vi "Push Sample.vi"(8 "error in (no error)":errorcluster, 11 "cRIO-CO2 in":refnum<class "cRIO-CO2.lvclass">) -> (0 "error out":errorcluster, 3 "cRIO-CO2 out":refnum<class "cRIO-CO2.lvclass">)   [LabVIEW 2015, in "cRIO-Carbondioxide.lvlib" / "cRIO-CO2.lvlib" / "cRIO-CO2.lvclass"]
uses:
  cRIO-CO2.lvclass
  cRIO-CO2.lvclass/cRIO-CO2.ctl
  Controls/Sample Push State Enumerator.ctl
  cRIO-CO2 Messages/Sample Push Reset to Idle Msg/Sample Push Reset to Idle Msg.lvclass/Sample Push Reset to Idle Msg.ctl
  <vilib>/ActorFramework/Message Enqueuer/Message Enqueuer.lvclass/Message Enqueuer.ctl
  Controls/Sample Transfer Container Enumerator.ctl
  Blowers Heaters Enumerator.ctl
  Controls/Sample Transfer State Enumerator.ctl
  <vilib>/ActorFramework/Time-Delayed Send Message/Time-Delay Override Options.ctl
  <vilib>/ActorFramework/Message Enqueuer/Enqueue.vi
  State Elapsed Time.vi
  <vilib>/ActorFramework/Message Priority Queue/Priority Enqueue.vi
  cRIO-CO2 Messages/Sample Push Reset to Idle Msg/Sample Push Reset to Idle Msg.lvclass
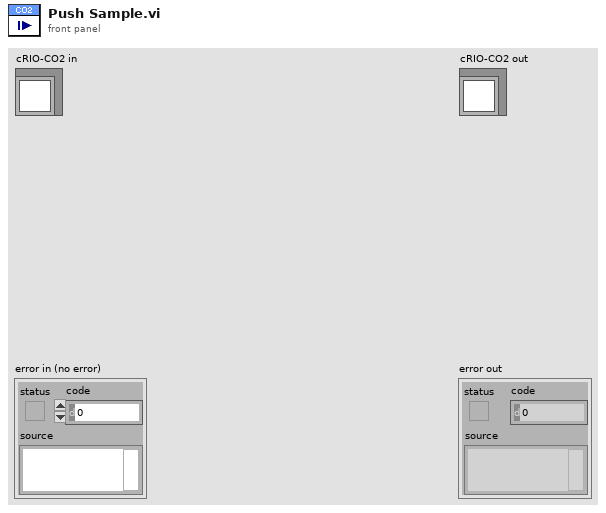
[diagram p1: front panel]
types:
  T1 = typedef "Sample Push State Enumerator.ctl" = enum16{"Undefined", "Initialize", "Dilute", "Close Transfer Line", "Start Heaters", "Warm Up Syringe", "Ready to Push", "Push", "Initiate Stash", "Stash", "Complete", "Abort", "Idle", "Error"}
  T2 = typedef "Sample Transfer Container Enumerator.ctl" = enum16{"None", "Sample 1", "Sample 2", "Sample 3", "Sample 4", "Sample 5", "Storage 01", "Storage 02", "Storage 03", "Storage 04", "Storage 05", "Storage 06", "Storage 07", "Storage 08", "Storage 09", "Storage 10", "Storage 11", "Storage 12", "Syringe", "Undefined"}
  T3 = typedef "cRIO-Carbondioxide.lvlib/cRIO-CO2.lvlib/cRIO-CO2.lvclass/Blowers Heaters Enumerator.ctl" = enum16{"Tank Blower 1", "Tank Blower 2", "Tank Blower 3", "Tank Blower 4", "Syringe Blower", "Syringe Heater", "Piston Heater", "Undefined"}
  T4 = typedef "Sample Transfer State Enumerator.ctl" = enum16{"Idle", "Initialize", "Check Containers", "Check Temperatures", "Start Turbo", "Warm Up Containers", "Prepare for purging", "Purge Capillary", "Purge", "Open Containers", "Introduce Sample", "Measure Base Pressure", "Home Syringe", "Start Freezer", "Freeze Target", "Crystalize", "Initiate Stash", "Stash", "Polish", "Stop Freezers", "Push Sample", "Complete", "Abort", "Error", "Undefined"}
  T5 = typedef "Time-Delay Override Options.ctl" = enum16{"Send next copy now", "Skip next scheduled copy", "Send next copy now and stop all further copies", "Stop all further copies"}
  T6 = typedef "Vacuum State Enumerator.ctl" = enum16{"Pressure Rising", "Plateau", "Pressure Dropping", "Valley", "Low Valley", "Leak", "Unknown"}
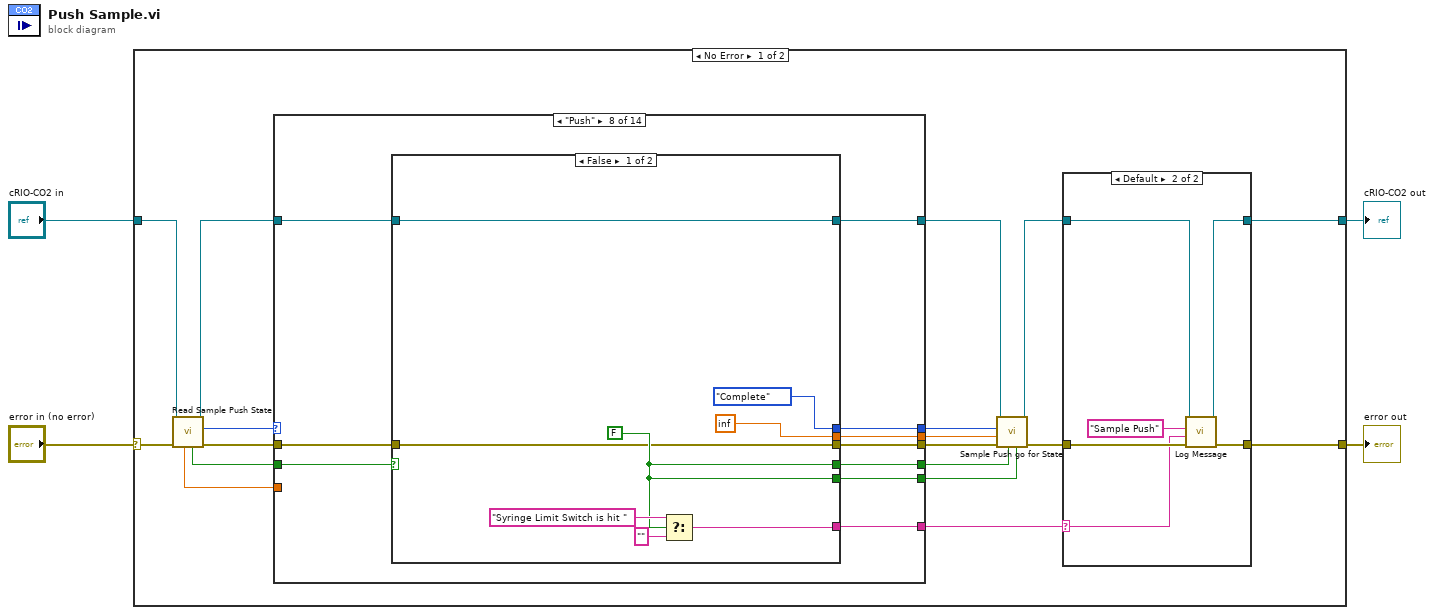
[diagram p0: block diagram]
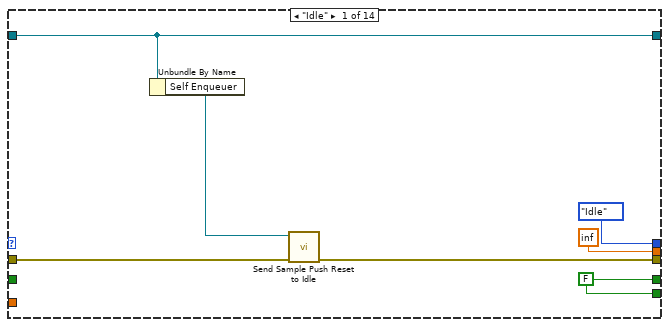
[diagram p3: hidden frame]
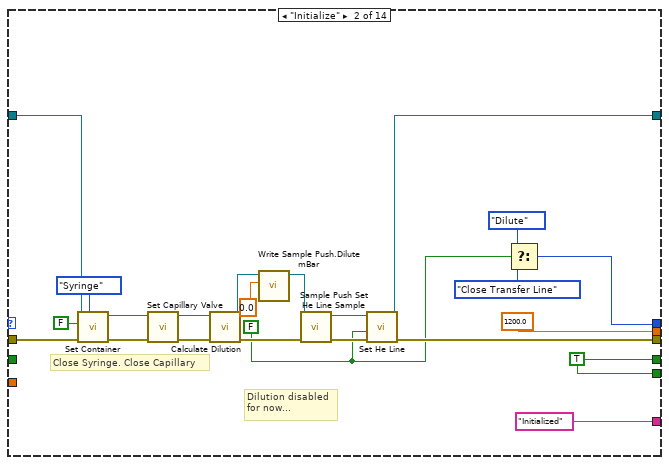
[diagram p4: hidden frame]
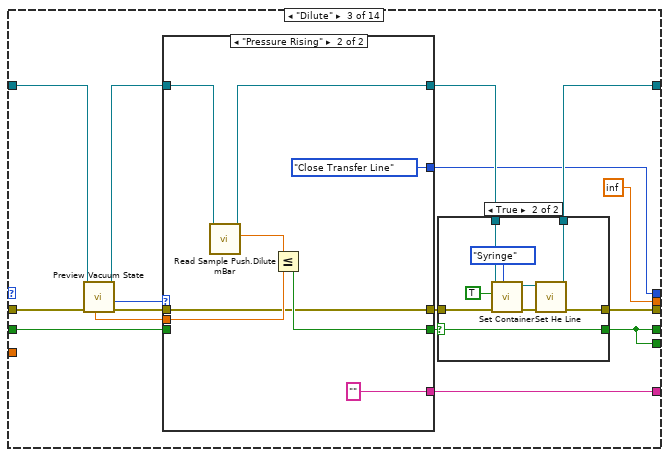
[diagram p5: hidden frame]
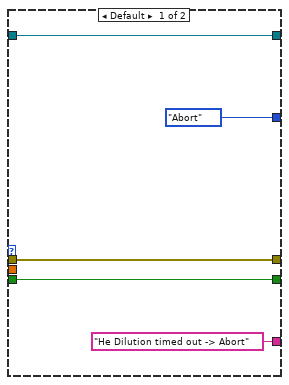
[diagram p7: hidden frame]
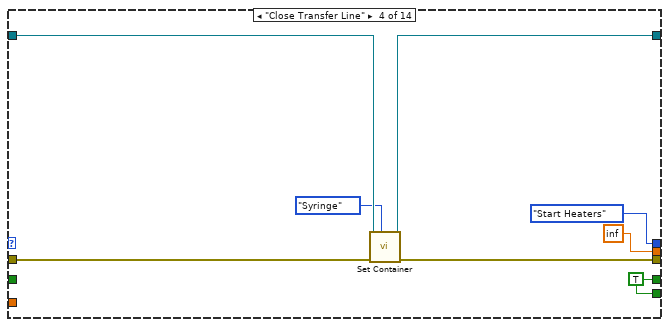
[diagram p8: hidden frame]
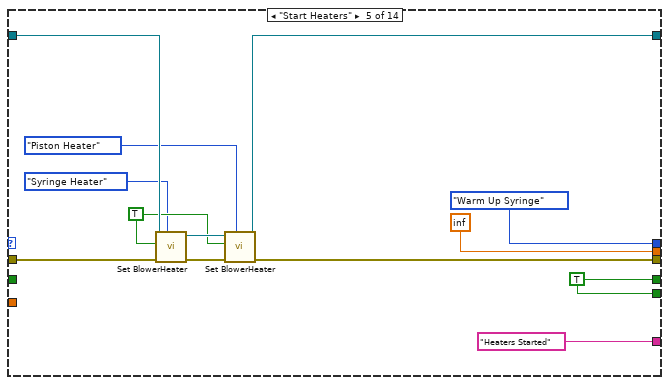
[diagram p9: hidden frame]
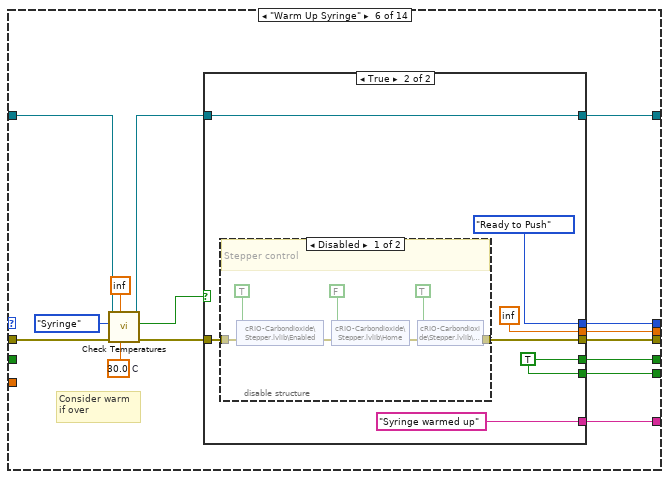
[diagram p10: hidden frame]
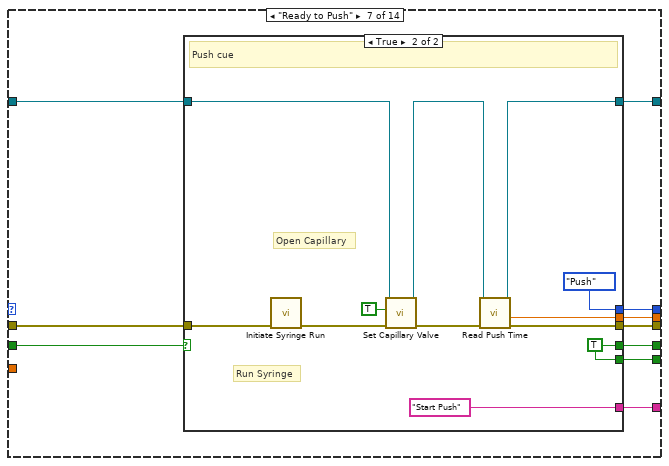
[diagram p13: hidden frame]
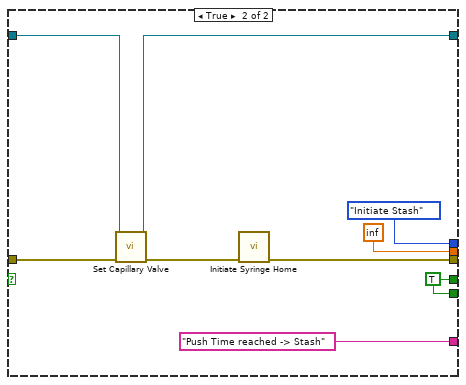
[diagram p15: hidden frame]
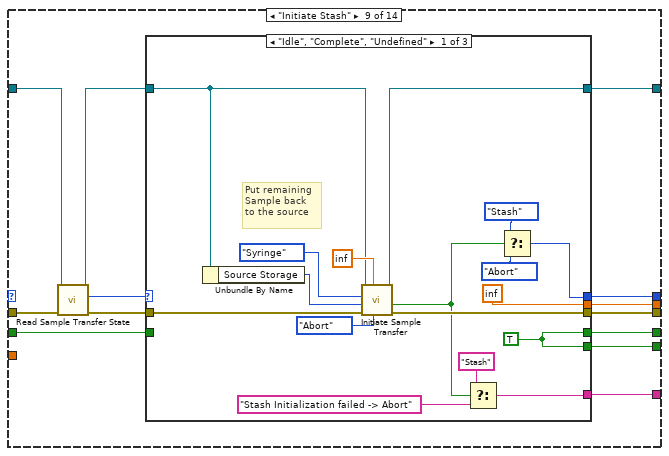
[diagram p16: hidden frame]
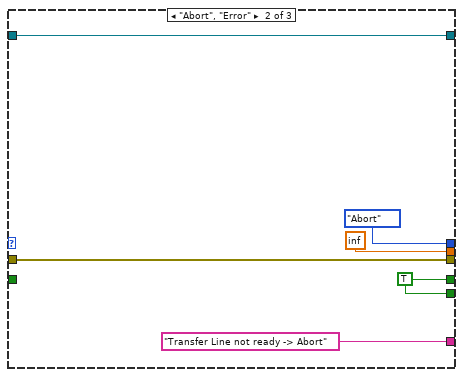
[diagram p17: hidden frame]
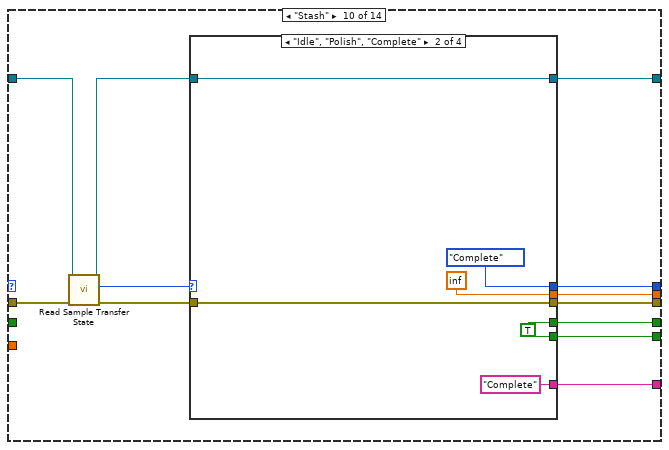
[diagram p19: hidden frame]
diagram:
  n1 = case shown="No Error" "error in (no error)" {
    selector: "error in (no error)" -> [w22 w326]
    tunnel: [w17 w326] -> w3
    tunnel: [w16 w325] -> w1
    tunnel: "cRIO-CO2 in" -> [w21 w325]
    frame No Error {
      n2 = call "Read Sample Push State.vi"("error in (no error)"=w22, "cRIO-CO2 in"=w21) -> ("error out"=w20:errorcluster, "Sample Push State"=w18:T1, "cRIO-CO2 out"=w19:refnum<class "cRIO-CO2.lvclass">, "Timeout?"=w14:bool, "Elapsed Time (s)"=w6:dbl)  [unwired: 3 in, 2 out]
      n3 = case shown="\"Push\"" w18 {
        tunnel: w20 -> [w34 w59 w75 w106 w122 w130 w155 w179 w218 w255 w287 w297 w308 w323]
        tunnel: [w31 w50 w67 w105 w112 w136 w162 w186 w213 w249 w277 w299 w314 w323] -> w13
        tunnel: w19 -> [w32 w57 w74 w104 w121 w126 w164 w188 w217 w254 w286 w296 w306 w324]
        tunnel: [_ "Initialized" ("String") w62 _ "Heaters Started" ("String") w135 w161 w185 w207 w244 "Complete" ("String") "Aborted" ("String") "Error" ("String") _] -> w15
        tunnel: w14 -> [_ _ w69 _ _ _ w156 w184 w206 _ _ _ _ _]
        tunnel: [w37 w54 w63 w107 w111 w132 w160 w183 w210 w246 w283 FALSE ("Publish? (T)") FALSE ("Publish? (T)") w321] -> w10
        tunnel: [w37 w54 w63 w107 w111 w131 w157 w180 w209 w245 w282 FALSE ("Publish? (T)") FALSE ("Publish? (T)") w321] -> w9
        tunnel: [Sample_Push_State_Enumerator."Idle" ("Sample Push State") w41 w61 Sample_Push_State_Enumerator."Start Heaters" ("Sample Push State") Sample_Push_State_Enumerator."Warm Up Syringe" ("Sample Push State") w133 w159 w182 w212 w248 Sample_Push_State_Enumerator."Idle" ("Sample Push State") Sample_Push_State_Enumerator."Idle" ("Sample Push State") Sample_Push_State_Enumerator."Idle" ("Sample Push State") Sample_Push_State_Enumerator."Idle" ("Sample Push State")] -> w8
        tunnel: [inf ("State Timeout (Inf=no timeout )") 1200.0 ("State Timeout (Inf=no timeout )") inf ("State Timeout (Inf=no timeout )") inf ("State Timeout (Inf=no timeout )") inf ("State Timeout (Inf=no timeout )") w134 w158 w181 w211 w247 inf ("State Timeout (Inf=no timeout )") inf ("State Timeout (Inf=no timeout )") inf ("State Timeout (Inf=no timeout )") inf ("State Timeout (Inf=no timeout )")] -> w7
        tunnel: w6 -> [_ _ _ _ _ _ _ _ _ _ _ _ _ _]
        tunnel: [w32 w49 w65 w103 w113 w137 w163 w187 w215 w252 w278 w298 w313 w324] -> w5
        frame "Idle" {
          w37 = FALSE ("Publish? (T)")
          n4 = Unbundle By Name(w32) -> ("Self Enqueuer"=w33:refnum<class "Message Enqueuer.lvclass">)
          n5 = call "Send Sample Push Reset to Idle.vi"("error in (no error)"=w34, "Message Enqueuer"=w33) -> ("error out"=w31:errorcluster)  [unwired: 8 in, 1 out]
        }
        frame "Initialize" {
          w39 = FALSE ("Open/Close (Close)")
          w54 = TRUE ("Publish? (T)")
          # "Dilution disabled\nfor now..."
          # "Close Syringe. Close Capillary"
          n6 = call "Set Container.vi"("Container"=Sample_Transfer_Container_Enumerator."Syringe", "error in (no error)"=w59, "Open/Close (Close)"=FALSE, "cRIO-CO2 in"=w57) -> ("error out"=w56:errorcluster, "cRIO-CO2 out"=w55:refnum<class "cRIO-CO2.lvclass">)  [unwired: 6 in]
          n7 = call "Set Capillary Valve.vi"("error in (no error)"=w56, "cRIO-CO2 in"=w55) -> ("error out"=w52:errorcluster, "cRIO-CO2 out"=w51:refnum<class "cRIO-CO2.lvclass">)  [unwired: 8 in]
          n8 = call "Calculate Dilution.vi"("error in (no error)"=w52, "cRIO-CO2 in"=w51) -> ("error out"=w47:errorcluster, "cRIO-CO2 out"=w48:refnum<class "cRIO-CO2.lvclass">)  [unwired: 6 in, 2 out]
          n9 = call "Write Sample Push.Dilute mBar.vi"("Dilute mBar"=0.0, "cRIO-CO2 in"=w48) -> ("cRIO-CO2 out"=w45:refnum<class "cRIO-CO2.lvclass">)  [unwired: 9 in]
          n10 = call "Sample Push Set He Line Sample.vi"("error in (no error)"=w47, "cRIO-CO2 in"=w45) -> ("error out"=w46:errorcluster, "cRIO-CO2 out"=w44:refnum<class "cRIO-CO2.lvclass">)  [unwired: 8 in]
          n11 = call "Set He Line.vi"("error in (no error)"=w46, "Open/Close (Close)"=w39, "cRIO-CO2 in"=w44) -> ("error out"=w50:errorcluster, "cRIO-CO2 out"=w49:refnum<class "cRIO-CO2.lvclass">)  [unwired: 7 in]
          n12 = Select(t=Sample_Push_State_Enumerator."Dilute" ("Sample Push State"), s=w39, f=Sample_Push_State_Enumerator."Close Transfer Line" ("Sample Push State")) -> (s? t:f=w41:T1)
        }
        frame "Dilute" {
          n13 = call "Preview Vacuum State.vi"("error in (no error)"=w75, "cRIO-CO2 in"=w74) -> ("error out"=w71:errorcluster, "State"=w73:T6, "cRIO-CO2 out"=w72:refnum<class "cRIO-CO2.lvclass">, "Raw Pressure"=w70:dbl)  [unwired: 3 in, 3 out]
          n14 = case shown="\"Pressure Rising\"" w73 {
            tunnel: w72 -> [w92 w99]
            tunnel: w71 -> [w93 w97]
            tunnel: w70 -> [_ w100]
            tunnel: w69 -> [w91 _]
            tunnel: [w93 w97] -> w68
            tunnel: [w91 w98] -> w64
            tunnel: [w92 w96] -> w66
            tunnel: ["He Dilution timed out -> Abort" ("String") "" ("String")] -> w62
            tunnel: [Sample_Push_State_Enumerator."Abort" ("Sample Push State") Sample_Push_State_Enumerator."Close Transfer Line" ("Sample Push State")] -> w61
            frame Default {
            }
            frame "Pressure Rising" {
              n15 = call "Read Sample Push.Dilute mBar.vi"("cRIO-CO2 in"=w99) -> ("Dilute mBar"=w101:dbl, "cRIO-CO2 out"=w96:refnum<class "cRIO-CO2.lvclass">)  [unwired: 9 in]
              n16 = Less Or Equal?(x=w101, y=w100) -> (x <= y?=w98:bool)
            }
          }
          n17 = case shown="True" w64 {
            selector: w64 -> [w78 w86]
            tunnel: w68 -> [w79 w85]
            tunnel: [w79 w88] -> w67
            tunnel: w66 -> [w77 w82]
            tunnel: [w77 w87] -> w65
            tunnel: [w78 w86] -> w63
            frame False {
            }
            frame True {
              n18 = call "Set Container.vi"("Container"=Sample_Transfer_Container_Enumerator."Syringe", "error in (no error)"=w85, "Open/Close (Close)"=TRUE, "cRIO-CO2 in"=w82) -> ("error out"=w84:errorcluster, "cRIO-CO2 out"=w83:refnum<class "cRIO-CO2.lvclass">)  [unwired: 6 in]
              n19 = call "Set He Line.vi"("error in (no error)"=w84, "cRIO-CO2 in"=w83) -> ("error out"=w88:errorcluster, "cRIO-CO2 out"=w87:refnum<class "cRIO-CO2.lvclass">)  [unwired: 8 in]
            }
          }
        }
        frame "Close Transfer Line" {
          w107 = TRUE ("Publish? (T)")
          n20 = call "Set Container.vi"("Container"=Sample_Transfer_Container_Enumerator."Syringe", "error in (no error)"=w106, "cRIO-CO2 in"=w104) -> ("error out"=w105:errorcluster, "cRIO-CO2 out"=w103:refnum<class "cRIO-CO2.lvclass">)  [unwired: 7 in]
        }
        frame "Start Heaters" {
          w111 = TRUE ("Publish? (T)")
          w118 = TRUE ("ON/OFF (OFF)")
          n21 = call "Set BlowerHeater.vi"("Blower/Heater"=Blowers_Heaters_Enumerator."Syringe Heater", "error in (no error)"=w122, "ON/OFF (OFF)"=w118, "cRIO-CO2 in"=w121) -> ("error out"=w120:errorcluster, "cRIO-CO2 out"=w119:refnum<class "cRIO-CO2.lvclass">)  [unwired: 6 in]
          n22 = call "Set BlowerHeater.vi"("Blower/Heater"=Blowers_Heaters_Enumerator."Piston Heater", "error in (no error)"=w120, "ON/OFF (OFF)"=w118, "cRIO-CO2 in"=w119) -> ("error out"=w112:errorcluster, "cRIO-CO2 out"=w113:refnum<class "cRIO-CO2.lvclass">)  [unwired: 6 in]
        }
        frame "Warm Up Syringe" {
          w128 = 30.0  # C
          # "Consider warm\nif over"
          n23 = call "Check Temperatures.vi"("lower limit (10C)"=w128, "upper limit (100C)"=inf, "error in (no error)"=w130, "Container"=Sample_Transfer_Container_Enumerator."Syringe", "cRIO-CO2 in"=w126) -> ("error out"=w129:errorcluster, "In Range?"=w124:bool, "cRIO-CO2 out"=w125:refnum<class "cRIO-CO2.lvclass">)  [unwired: 4 in]
          n24 = case shown="True" w124 {
            tunnel: w125 -> [w139 w143]
            tunnel: [w139 w143] -> w137
            tunnel: w129 -> [w138 w145]
            tunnel: [w138 w144] -> w136
            tunnel: [_ "Syringe warmed up"] -> w135
            tunnel: [_ inf ("State Timeout (Inf=no timeout )")] -> w134
            tunnel: [_ Sample_Push_State_Enumerator."Ready to Push" ("Sample Push State")] -> w133
            tunnel: [_ w141] -> w132
            tunnel: [_ w141] -> w131
            frame False {
            }
            frame True {
              w141 = TRUE
              n25 = disable-structure shown="Disabled" {
                disable-tunnel: w145 -> [w153 w154]
                disable-tunnel: [w151 w154] -> w144
                frame Disabled {
                  # "Stepper control"
                  n26 = shared-variable "cRIO-Carbondioxide\\Stepper.lvlib\\Enabled"(TRUE ("Enabled"), error in=w153) -> (error out=w150:errorcluster)
                  n27 = shared-variable "cRIO-Carbondioxide\\Stepper.lvlib\\Home"(FALSE ("Home"), error in=w150) -> (error out=w149:errorcluster)
                  n28 = shared-variable "cRIO-Carbondioxide\\Stepper.lvlib\\Run"(TRUE ("Run"), error in=w149) -> (error out=w151:errorcluster)
                }
                frame Enabled {
                }
              }
            }
          }
        }
        frame "Ready to Push" {
          n29 = case shown="True" w156 {
            tunnel: w164 -> [w166 w175]
            tunnel: [w166 w167] -> w163
            tunnel: [w165 w170] -> w162
            tunnel: [_ "Start Push"] -> w161
            tunnel: w155 -> [w165 w173]
            tunnel: [_ w176] -> w160
            tunnel: [_ Sample_Push_State_Enumerator."Push" ("Sample Push State")] -> w159
            tunnel: [_ w169] -> w158
            tunnel: [_ w176] -> w157
            frame False {
              # "Waiting for the Push Cue (Timeout cleared)"
            }
            frame True {
              w176 = TRUE ("Timeout?")
              # "Run Syringe"
              # "Open Capillary"
              # "Push cue"
              n30 = call "Initiate Syringe Run.vi"("error in (no error)"=w173) -> ("error out"=w172:errorcluster)  [unwired: 10 in]
              n31 = call "Set Capillary Valve.vi"("error in (no error)"=w172, "ON/OFF(OFF)"=TRUE, "cRIO-CO2 in"=w175) -> ("error out"=w171:errorcluster, "cRIO-CO2 out"=w168:refnum<class "cRIO-CO2.lvclass">)  [unwired: 7 in]
              n32 = call "Read Push Time.vi"("error in (no error)"=w171, "cRIO-CO2 in"=w168) -> ("error out"=w170:errorcluster, "Push Time (sec)"=w169:dbl, "cRIO-CO2 out"=w167:refnum<class "cRIO-CO2.lvclass">)  [unwired: 7 in]
            }
          }
        }
        frame "Push" {
          n33 = case shown="False" w184 {
            tunnel: w188 -> [w196 w200]
            tunnel: [w196 w199] -> w187
            tunnel: [w189 w197] -> w186
            tunnel: [w193 "Push Time reached -> Stash"] -> w185
            tunnel: w179 -> [w189 w201]
            tunnel: [w190 w204] -> w183
            tunnel: [Sample_Push_State_Enumerator."Complete" ("Sample Push State") Sample_Push_State_Enumerator."Initiate Stash" ("Sample Push State")] -> w182
            tunnel: [inf inf] -> w181
            tunnel: [w190 w204] -> w180
            frame False {
              w190 = FALSE
              n34 = Select(t="Syringe Limit Switch is hit ", s=w190, f="") -> (s? t:f=w193:string)
            }
            frame True {
              w204 = TRUE ("Timeout?")
              n35 = call "Set Capillary Valve.vi"("error in (no error)"=w201, "cRIO-CO2 in"=w200) -> ("error out"=w198:errorcluster, "cRIO-CO2 out"=w199:refnum<class "cRIO-CO2.lvclass">)  [unwired: 8 in]
              n36 = call "Initiate Syringe Home.vi"("error in (no error)"=w198) -> ("error out"=w197:errorcluster)  [unwired: 10 in]
            }
          }
        }
        frame "Initiate Stash" {
          n37 = call "Read Sample Transfer State.vi"("error in (no error)"=w218, "cRIO-CO2 in"=w217) -> ("error out"=w214:errorcluster, "Sample Transfer State"=w208:T4, "cRIO-CO2 out"=w216:refnum<class "cRIO-CO2.lvclass">)  [unwired: 4 in, 3 out]
          n38 = case shown="\"Idle\", \"Complete\", \"Undefined\"" w208 {
            tunnel: w216 -> [w231 w241 w243]
            tunnel: [w233 w241 w243] -> w215
            tunnel: w214 -> [w234 w240 w242]
            tunnel: [w228 w240 w242] -> w213
            tunnel: [w223 Sample_Push_State_Enumerator."Abort" ("Sample Push State") _] -> w212
            tunnel: [inf ("State Timeout (Inf=no timeout )") inf ("State Timeout (Inf=no timeout )") _] -> w211
            tunnel: [w227 w237 _] -> w210
            tunnel: [w227 w237 _] -> w209
            tunnel: [w222 "Transfer Line not ready -> Abort" _] -> w207
            tunnel: w206 -> [_ _ _]
            frame "Idle", "Complete", "Undefined" {
              w227 = TRUE
              # "Put remaining\nSample back\nto the source"
              n39 = Unbundle By Name(w231) -> ("Source Storage"=w229:T2)
              n40 = call "Initiate Sample Transfer.vi"("Fail State (Idle)"=Sample_Transfer_State_Enumerator."Abort", "Transfer mBar"=inf, "error in (no error)"=w234, "Target Container"=w229, "Source Container"=Sample_Transfer_Container_Enumerator."Syringe", "cRIO-CO2 in"=w231) -> ("error out"=w228:errorcluster, "Success?"=w220:bool, "cRIO-CO2 out"=w233:refnum<class "cRIO-CO2.lvclass">)  [unwired: 3 in]
              n41 = Select(t="Stash", s=w220, f="Stash Initialization failed -> Abort" ("t")) -> (s? t:f=w222:string)
              n42 = Select(t=Sample_Push_State_Enumerator."Stash", s=w220, f=Sample_Push_State_Enumerator."Abort" ("Sample Push State")) -> (s? t:f=w223:T1)
            }
            frame "Abort", "Error" {
              w237 = TRUE
            }
            frame Default {
            }
          }
        }
        frame "Stash" {
          n43 = call "Read Sample Transfer State.vi"("error in (no error)"=w255, "cRIO-CO2 in"=w254) -> ("error out"=w250:errorcluster, "Sample Transfer State"=w253:T4, "cRIO-CO2 out"=w251:refnum<class "cRIO-CO2.lvclass">)  [unwired: 4 in, 3 out]
          n44 = case shown="\"Idle\", \"Polish\", \"Complete\"" w253 {
            tunnel: [w257 w263 w269 w275] -> w252
            tunnel: w251 -> [w257 w263 w269 w275]
            tunnel: w250 -> [w256 w258 w268 w274]
            tunnel: [w256 w258 w268 w274] -> w249
            tunnel: [_ Sample_Push_State_Enumerator."Complete" ("Sample Push State") Sample_Push_State_Enumerator."Abort" ("Sample Push State") Sample_Push_State_Enumerator."Abort" ("Sample Push State")] -> w248
            tunnel: [_ inf inf inf] -> w247
            tunnel: [_ w260 w265 w271] -> w246
            tunnel: [_ w260 w265 w271] -> w245
            tunnel: [_ "Complete" "Transfer Error -> Abort" "Transfer Aborted -> Abort"] -> w244
            frame Default {
            }
            frame "Idle", "Polish", "Complete" {
              w260 = TRUE
            }
            frame "Error" {
              w265 = TRUE
            }
            frame "Abort" {
              w271 = TRUE
            }
          }
        }
        frame "Complete" {
          w282 = FALSE  # Publish
          w283 = FALSE  # Go For State
          # "Close Capillary"
          n45 = call "Set Capillary Valve.vi"("error in (no error)"=w287, "cRIO-CO2 in"=w286) -> ("error out"=w280:errorcluster, "cRIO-CO2 out"=w279:refnum<class "cRIO-CO2.lvclass">)  [unwired: 8 in]
          n46 = call "Send Sample Push Notification.vi"("notification (Send next copy now)"=Time-Delay_Override_Options."Stop all further copies", "error in (no error)"=w280, "cRIO-CO2 in"=w279) -> ("error out"=w277:errorcluster, "cRIO-CO2 out"=w278:refnum<class "cRIO-CO2.lvclass">)  [unwired: 7 in]
        }
        frame "Abort" {
          # "Close Syringe Line and Capillary"
          n47 = call "Set Container.vi"("Container"=Sample_Transfer_Container_Enumerator."Syringe", "error in (no error)"=w297, "cRIO-CO2 in"=w296) -> ("error out"=w294:errorcluster, "cRIO-CO2 out"=w293:refnum<class "cRIO-CO2.lvclass">)  [unwired: 7 in]
          n48 = call "Set Capillary Valve.vi"("error in (no error)"=w294, "cRIO-CO2 in"=w293) -> ("error out"=w290:errorcluster, "cRIO-CO2 out"=w291:refnum<class "cRIO-CO2.lvclass">)  [unwired: 8 in]
          n49 = call "Set He Line.vi"("error in (no error)"=w290, "cRIO-CO2 in"=w291) -> ("error out"=w288:errorcluster, "cRIO-CO2 out"=w289:refnum<class "cRIO-CO2.lvclass">)  [unwired: 8 in]
          n50 = call "Send Sample Push Notification.vi"("notification (Send next copy now)"=Time-Delay_Override_Options."Stop all further copies", "error in (no error)"=w288, "cRIO-CO2 in"=w289) -> ("error out"=w299:errorcluster, "cRIO-CO2 out"=w298:refnum<class "cRIO-CO2.lvclass">)  [unwired: 7 in]
        }
        frame "Error" {
          # "Close Syringe Line and Capillary"
          n51 = call "Set Container.vi"("Container"=Sample_Transfer_Container_Enumerator."Syringe", "error in (no error)"=w308, "cRIO-CO2 in"=w306) -> ("error out"=w310:errorcluster, "cRIO-CO2 out"=w309:refnum<class "cRIO-CO2.lvclass">)  [unwired: 7 in]
          n52 = call "Set Capillary Valve.vi"("error in (no error)"=w310, "cRIO-CO2 in"=w309) -> ("error out"=w307:errorcluster, "cRIO-CO2 out"=w305:refnum<class "cRIO-CO2.lvclass">)  [unwired: 8 in]
          n53 = call "Send Sample Push Notification.vi"("notification (Send next copy now)"=Time-Delay_Override_Options."Stop all further copies", "error in (no error)"=w307, "cRIO-CO2 in"=w305) -> ("error out"=w314:errorcluster, "cRIO-CO2 out"=w313:refnum<class "cRIO-CO2.lvclass">)  [unwired: 7 in]
        }
        frame "Undefined" {
          w321 = TRUE ("Publish? (T)")
        }
      }
      n54 = call "Sample Push go for State.vi"("Publish? (T)"=w9, "Really? (T)"=w10, "error in (no error)"=w13, "State Timeout (Inf=no timeout )"=w7, "Sample Push State"=w8, "cRIO-CO2 in"=w5) -> ("error out"=w12:errorcluster, "cRIO-CO2 out"=w11:refnum<class "cRIO-CO2.lvclass">)  [unwired: 4 in]
      n55 = case shown="Default" w15 {
        selector: w15 -> [_ w25]
        tunnel: w12 -> [w23 w30]
        tunnel: [w23 w29] -> w17
        tunnel: w11 -> [w24 w28]
        tunnel: [w24 w27] -> w16
        frame "" {
        }
        frame Default {
          n56 = call "Log Message.vi"("error in (no error)"=w30, "String"=w25, "Source Name"="Sample Push", "cRIO-CO2 in"=w28) -> ("error out"=w29:errorcluster, "cRIO-CO2 out"=w27:refnum<class "cRIO-CO2.lvclass">)  [unwired: 6 in]
        }
      }
    }
    frame Error {
    }
  }
  "error out" <- w3
  "cRIO-CO2 out" <- w1
